vi "Reset With Defaults.vi"(8 "error in (no error)":errorcluster {"code" format="%.0x"}, 11 "instrument handle":refnum<k15>) -> (0 "error out":errorcluster {"code" format="%.0x"}, 3 "instrument handle out":refnum<k15>)   [LabVIEW 2014, in "Agilent NA.lvlib"]
doc: "Does the equivalent of Reset and then, (1) disables class extension capability groups, (2) sets properties to initial values defined by class specs, and (3) configures the driver to option string settings used when Initialize was last executed."
uses:
  Agilent NA.lvlib
  AgNA.dll
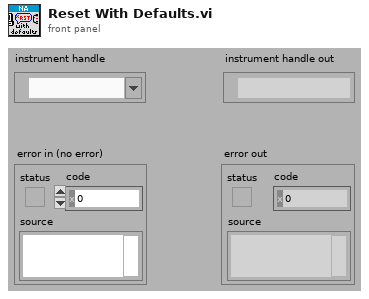
[diagram p1: front panel]
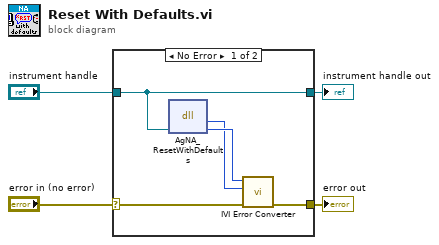
[diagram p0: block diagram]
diagram:
  n1 = case shown="No Error" "error in (no error)" {
    selector: "error in (no error)" -> [w5 w10]
    tunnel: [w6 w10] -> w4
    tunnel: "instrument handle" -> [w7 w11]
    tunnel: [w7 w11] -> w2
    frame No Error {
      n2 = dll-call lib="AgNA**.dll" fn="AgNA_ResetWithDefaults" ("LabVIEW:IviDmm_ResetWithDefaults")("instrument handle"=w7) -> ("Status"=w8:i32, "instrument handle"=w9:u32)  [unwired: 3 in, 2 out]
      n3 = call "IVI Error Converter.vi"("error in (no error)"=w5, "IVI error code (0)"=w8, "instrument handle"=w9) -> ("error out"=w6:errorcluster)  [unwired: 7 in, 1 out]
    }
    frame Error {
    }
  }
  "error out" <- w4
  "instrument handle out" <- w2
